vi "CONFIG (SubVI).vi"(10 "NewVal":enum16{"input", "output", "disable"}(ring), 11 "Enum in":refnum<vi>) -> (3 "String":string)   [LabVIEW 2017]
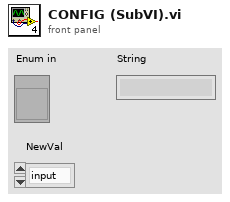
[diagram p1: front panel]
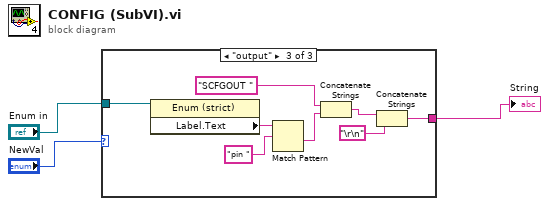
[diagram p0: block diagram]
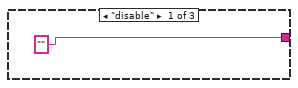
[diagram p2: hidden frame]
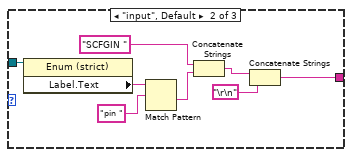
[diagram p3: hidden frame]
diagram:
  n1 = case shown="\"output\"" "NewVal" {
    tunnel: "Enum in" -> [_ w6 w13]
    tunnel: ["" w5 w14] -> w3
    frame "disable" {
    }
    frame "input", Default {
      n2 = property class="Enum (strict)"(reference=w6) -> ("Label.Text"=w11:string)  [unwired: 1 in, 2 out]
      n3 = Match Pattern(string=w11, regular expression="pin ") -> (after substring=w12:string)  [unwired: 1 in, 3 out]
      n4 = Concatenate Strings("SCFGIN " ("String 2"), w12) -> (w10:string)
      n5 = Concatenate Strings(w10, "\r\n") -> (w5:string)
    }
    frame "output" {
      n6 = property class="Enum (strict)"(reference=w13) -> ("Label.Text"=w19:string)  [unwired: 1 in, 2 out]
      n7 = Match Pattern(string=w19, regular expression="pin ") -> (after substring=w20:string)  [unwired: 1 in, 3 out]
      n8 = Concatenate Strings("SCFGOUT " ("String 2"), w20) -> (w18:string)
      n9 = Concatenate Strings(w18, "\r\n") -> (w14:string)
    }
  }
  "String" <- w3
